vi "Pulse RFmx.vi"(8 "error in":errorcluster, 11 "RFmx Settings":T1={"Center Frequency (Hz)"=10000000000.0, "Measurement Bandwidth (Hz)"=80000000.0, "Reference Level (dBm)"=10.0, "RFmx De-embedding"={"RFmx Name"="5842_0", "RFmx Port"="", "Attenuation"={"Mode"=enum."Constant Attenuation", "Constant Attenuation"={"RFmx External Attenuation (dB)"=1.2}, "s2p File"={"RFmx S-Parameters Orientation"=24000, "RFmx Attenuation s2p Path Name"="", "RFmx Attenuation s2p File"=path ""}}}, "Acquisition Length (s)"=0.0} {"RFmx De-embedding"."Attenuation"."s2p File"."RFmx S-Parameters Orientation" items=["Port1 Towards DUT"=24000, "Port2 Towards DUT"=24001]; "RFmx De-embedding"."Attenuation"."Constant Attenuation"."RFmx External Attenuation (dB)" format="%.2f"; "Reference Level (dBm)" format="%.2f"; "Measurement Bandwidth (Hz)" format="%.3p"; "Center Frequency (Hz)" format="%.6p"}) -> (0 "error out":errorcluster, 3 "RFmx session out":refnum<k21>)   [LabVIEW 2023]
uses:
  Controls/RFmx Config - Pulse.ctl
  FPT Shared VIs/De-embedding/RFmx Config.ctl
  <vilib>/RFmx/Pulse/mx/RFmxPulse.llb/RFmxPulse Select Measurement (Single).vi
  <resource>/objmgr/RFmxInstr.rc
  <resource>/objmgr/RFmxPulse.rc
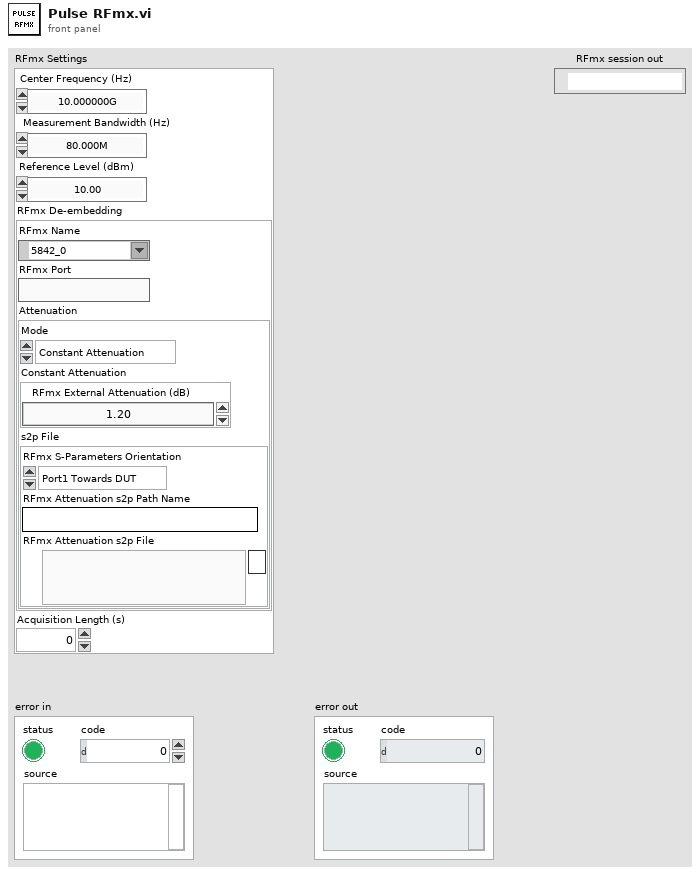
[diagram p1: front panel]
types:
  T1 = typedef "RFmx Config - Pulse.ctl" = cluster{"Center Frequency (Hz)":dbl, "Measurement Bandwidth (Hz)":dbl, "Reference Level (dBm)":dbl, "RFmx De-embedding":T2, "Acquisition Length (s)":dbl}
  T2 = typedef "RFmx Config.ctl" = cluster{"RFmx Name":refnum<k15>, "RFmx Port":string, "Attenuation":cluster{"Mode":enum32{"<None>", "Constant Attenuation", "s2p File"}, "Constant Attenuation":cluster{"RFmx External Attenuation (dB)":dbl}, "s2p File":cluster{"RFmx S-Parameters Orientation":i32, "RFmx Attenuation s2p Path Name":string, "RFmx Attenuation s2p File":path}}}
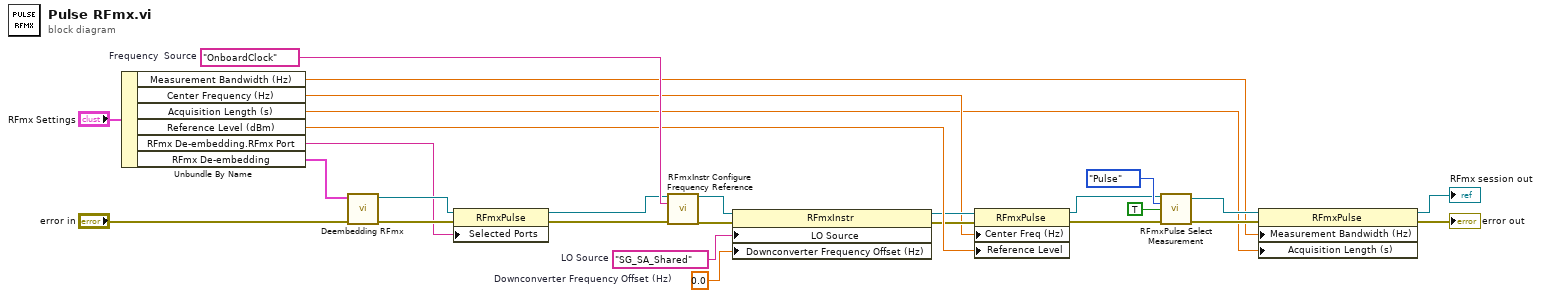
[diagram p0: block diagram]
diagram:
  w20 = "SG_SA_Shared"  # LO Source
  w19 = 0.0  # Downconverter Frequency Offset (Hz)
  w27 = "OnboardClock"  # Frequency  Source
  n1 = Unbundle By Name("RFmx Settings") -> ("Measurement Bandwidth (Hz)"=w9:dbl, "Center Frequency (Hz)"=w15:dbl, "Acquisition Length (s)"=w10:dbl, "Reference Level (dBm)"=w18:dbl, "RFmx De-embedding.RFmx Port"=w1:string, "RFmx De-embedding"=w11:T2)
  n2 = call "Deembedding RFmx.vi"("error in"="error in", "RFmx Settings"=w11) -> ("error out"=w3:errorcluster, "Refnum out"=w5:refnum<k21>)  [unwired: 8 in]
  n3 = property class="RFmxPulse"(reference=w5, error in=w3, "Selected Ports"=w1) -> (reference out=w4:refnum<k21>, error out=w2:errorcluster)
  n4 = call <vilib>:"RFmxInstr Configure Frequency Reference.vi"("Instrument Handle In"=w4, "Frequency Reference Source"=w27, "error in (no error)"=w2) -> ("Instrument Handle Out"=w22:refnum<k21>, "error out"=w21:errorcluster)  [unwired: 11 in]
  n5 = property class="RFmxInstr"(reference=w22, error in=w21, "LO Source"=w20, "Downconverter Frequency Offset (Hz)"=w19) -> (reference out=w17:refnum<k21>, error out=w16:errorcluster)
  n6 = property class="RFmxPulse"(reference=w17, error in=w16, "Center Freq (Hz)"=w15, "Reference Level"=w18) -> (reference out=w13:refnum<k21>, error out=w14:errorcluster)
  n7 = call-poly <vilib>:"RFmxPulse Select Measurement.vi"("Instrument Handle In"=w13, "Measurement"=enum16{"Pulse"}."Pulse", "Enable All Traces"=TRUE, "error in (no error)"=w14) -> ("Instrument Handle Out"=w24:refnum<k21>, "error out"=w23:errorcluster)  [unwired: 10 in]
  n8 = property class="RFmxPulse"(reference=w24, error in=w23, "Measurement Bandwidth (Hz)"=w9, "Acquisition Length (s)"=w10) -> (reference out=→"RFmx session out":refnum<k21>, error out=→"error out":errorcluster)
